vi "Buffer Make Buffer.vi"(5 "Capacity (1)":u32=1, 7 "Channel (Channel A)":T1, 8 "error in (no error)":errorcluster, 9 "Buffer Name (buf)":string="buf", 10 "Node In":string, 11 "VISA resource name":refnum<visa-resource-name>) -> (0 "error out":errorcluster, 2 "Node Out":string, 3 "VISA resource name out":refnum<visa-resource-name>, 4 "Command String":string)   [LabVIEW 2012, in "Keithley 2600 Series.lvlib"]
doc: "This VI will create a reading buffer in the instrument's volatile memory. This buffer will remain until it is either deleted by the user or the instrument is powered down.\n\n<b>Functions and Attributes Used</b>\nsmuX.makebuffer(buffersize)"
uses:
  Keithley 2600 Series.lvlib
  Private/GlobalVariables.vi
  Channel.ctl
panel:
  # "(c) 2008 Keithley Instruments, Inc.  ALL RIGHTS RESERVED."
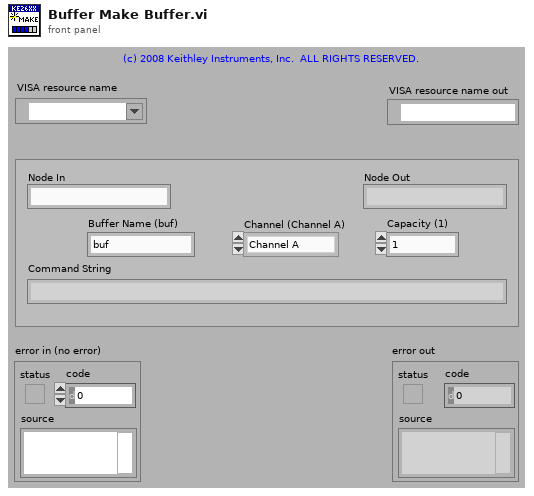
[diagram p1: front panel]
types:
  T1 = typedef "Keithley 2600 Series.lvlib/Channel.ctl" = enum32{"Channel A", "Channel B"}
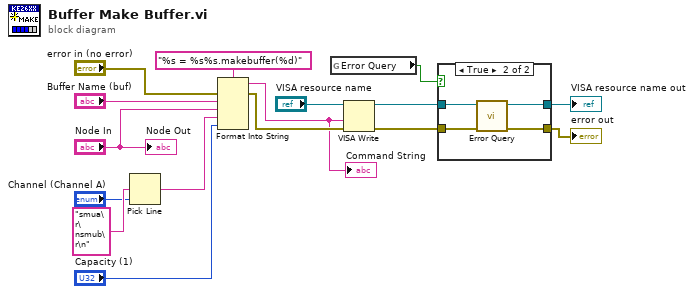
[diagram p0: block diagram]
diagram:
  n1 = Pick Line(multi-line string="smua\r\nsmub\r\n" ("options"), line index="Channel (Channel A)") -> (output string=w6:string)  [unwired: 1 out]
  n2 = Format Into String(format string="%s = %s%s.makebuffer(%d)", error in="error in (no error)", "Buffer Name (buf)", "Node In", w6, "Capacity (1)") -> (resulting string=w1:string, error out=w2:errorcluster)  [unwired: 1 in]
  "Command String" <- w1
  n3 = global read "GlobalVariables.vi" "Error Query"() -> (w14:bool)
  n4 = VISA Write(VISA resource name="VISA resource name", write buffer=w1, error in (no error)=w2) -> (VISA resource name out=w13:refnum<visa-resource-name>, error out=w12:errorcluster)  [unwired: 1 out]
  n5 = case shown="True" w14 {
    tunnel: w13 -> [w18 w22]
    tunnel: w12 -> [w17 w21]
    tunnel: [w18 w20] -> w11
    tunnel: [w17 w19] -> w10
    frame False {
    }
    frame True {
      n6 = call "Error Query.vi"("error in (no error)"=w21, "VISA resource name"=w22) -> ("error out"=w19:errorcluster, "VISA resource name out"=w20:refnum<visa-resource-name>)  [unwired: 8 out]
    }
  }
  "VISA resource name out" <- w11
  "error out" <- w10
  "Node Out" <- "Node In"
